vi "HoppingStep(Nonlinear-XZ-TargetModulation).vi"() -> ()   [LabVIEW 2014]
uses:
  <vilib>/Platform/TimedLoop/XDataNode/timing_clust.ctl
  <vilib>/Platform/TimedLoop/XDataNode/nitl_modes.ctl
  <vilib>/Platform/TimedLoop/XDataNode/wakeup.ctl
  <vilib>/rvi/Emulation/niFpgaGetClockAttributes.vi
  <vilib>/rvi/Emulation/niFpgaSctlEmulationGetInTimedLoop.vi
  <vilib>/rvi/Emulation/niFpgaEmulationReportErrorSimple.vi
  <vilib>/rvi/Emulation/niFpgaProcessEmulError.vi
  <vilib>/rvi/eio/common/nirviEmuTemplateMethod_errors.vi
  <vilib>/rvi/Emulation/niFpgaCriticalErrorInLSC.vi
  <vilib>/rvi/interface/RandomDataEmulation/niFpgaRandomDataHandleErrors.vi
  <vilib>/eio/EIONode/EIONode.xnode
  <vilib>/Platform/TimedLoop/XDataNode/XDataNode.xnode
  <vilib>/rvi/DataTransferAndStorage/Container/XNode/niFpgaContainer.xnode
  <vilib>/rvi/interface/RandomDataEmulation/nirviRandomDataFpgaReadWriteTemplate.vi
  <vilib>/Platform/TimedLoop/XDataNode/XDNodeRunTimeDep.lvlib
panel:
  in  "threshold":sgl
  in  "ExtraStepIn":u32
  in  "TimeConstant":u32
  in  "LowPassFilter":i16
  in  "BottomSleep us":i16=80
  in  "UpperSleep us":i16=150
  out "ZRealPos":i16
  in  "RelativeWithdraw":i16
  out "Waveform Chart":i32(graph)
  in  "stop":bool
  out "Z":i32(graph)
  in  "ZOffset":i16
  in  "XOffset":i16
  in  "XNum":i16
  in  "XStepIndex":i16
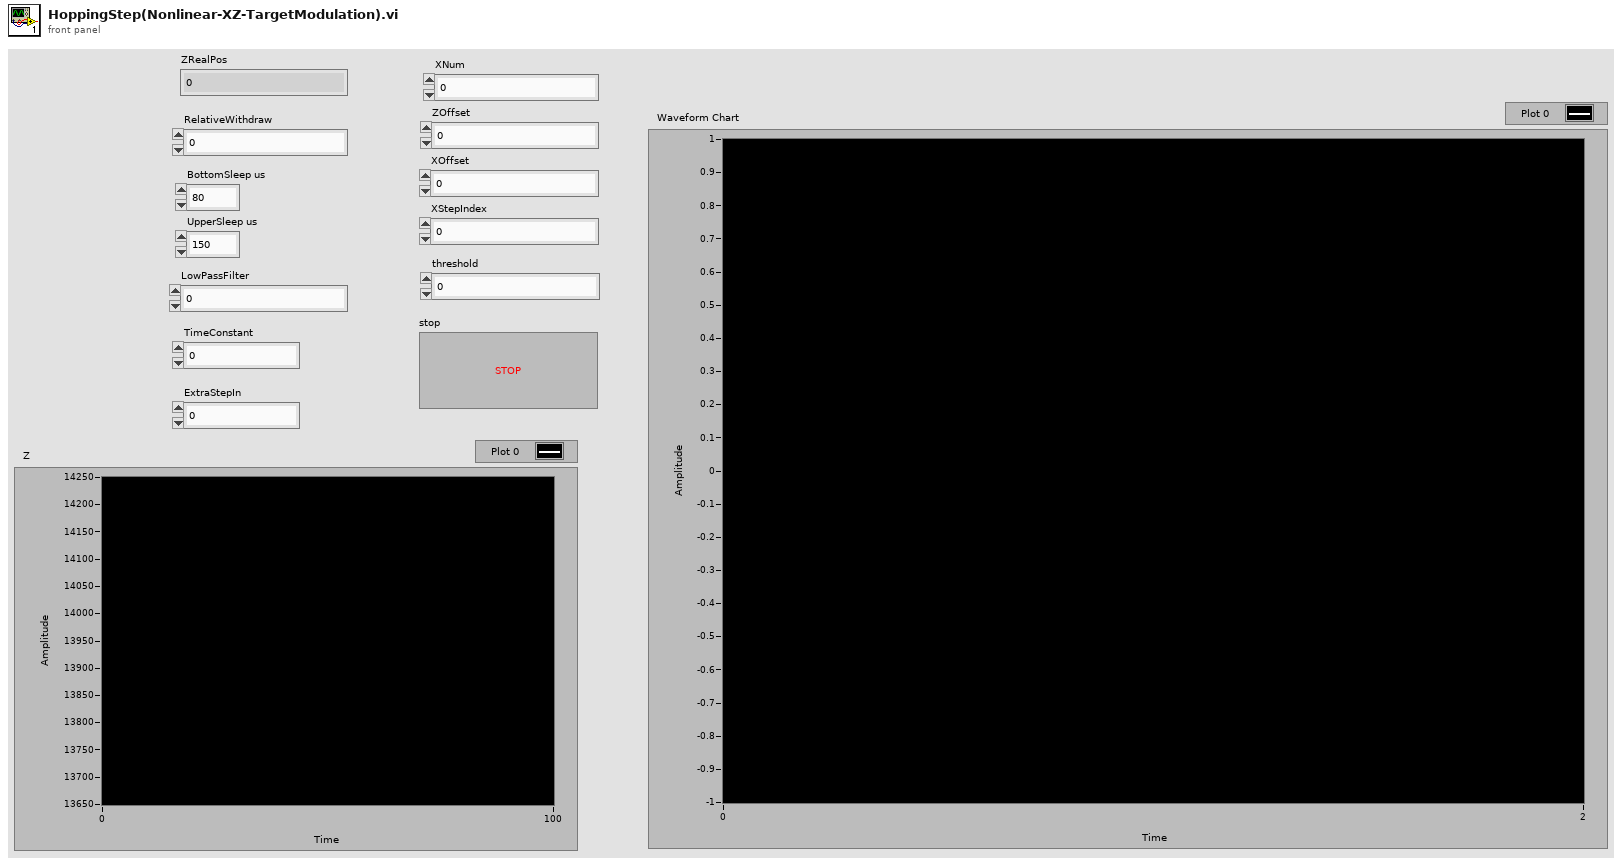
[diagram p1: front panel]
types:
  T1 = typedef "XDNodeRunTimeDep.lvlib/timing_clust.ctl" = cluster{"Expected End [f-1]":u64, "Actual End [f-1]":u64, "Finished Late? [f-1]":bool, "Expected End [i-1]":u64, "Actual End [i-1]":u64, "Finished Late? [i-1]":bool, "Expected Start [i]":u64, "Actual Start [i]":u64, "Expected Start [f]":u64, "Actual Start [f]":u64, "Source Name":string, "Structure Name":string, "Period":i64, "Deadline":i64, "Offset":i64, "Start":i64, "Priority":i32, "Timeout":i32, "Mode":T2, "Wakeup Reason":T3, "Error":errorcluster, "Source Type":string, "Secondary Source Type":string, "Global End Time":u64, "Global Start Time":u64, "Frame Duration":u64, "Iteration Duration":u64, "Assigned CPU":i32, "I/O Scan Engine Mode":u32}
  T2 = typedef "XDNodeRunTimeDep.lvlib/nitl_modes.ctl" = enum32{"No Change", "Process missed periods, maintain original phase", "Discard missed periods, maintain original phase", "Process missed periods, ignore original phase", "Discard missed periods, ignore original phase"}
  T3 = typedef "XDNodeRunTimeDep.lvlib/wakeup.ctl" = enum32{"Normal", "Aborted", "Asynchronous wakeup", "Timing source error", "Timed loop error", "Timeout"}
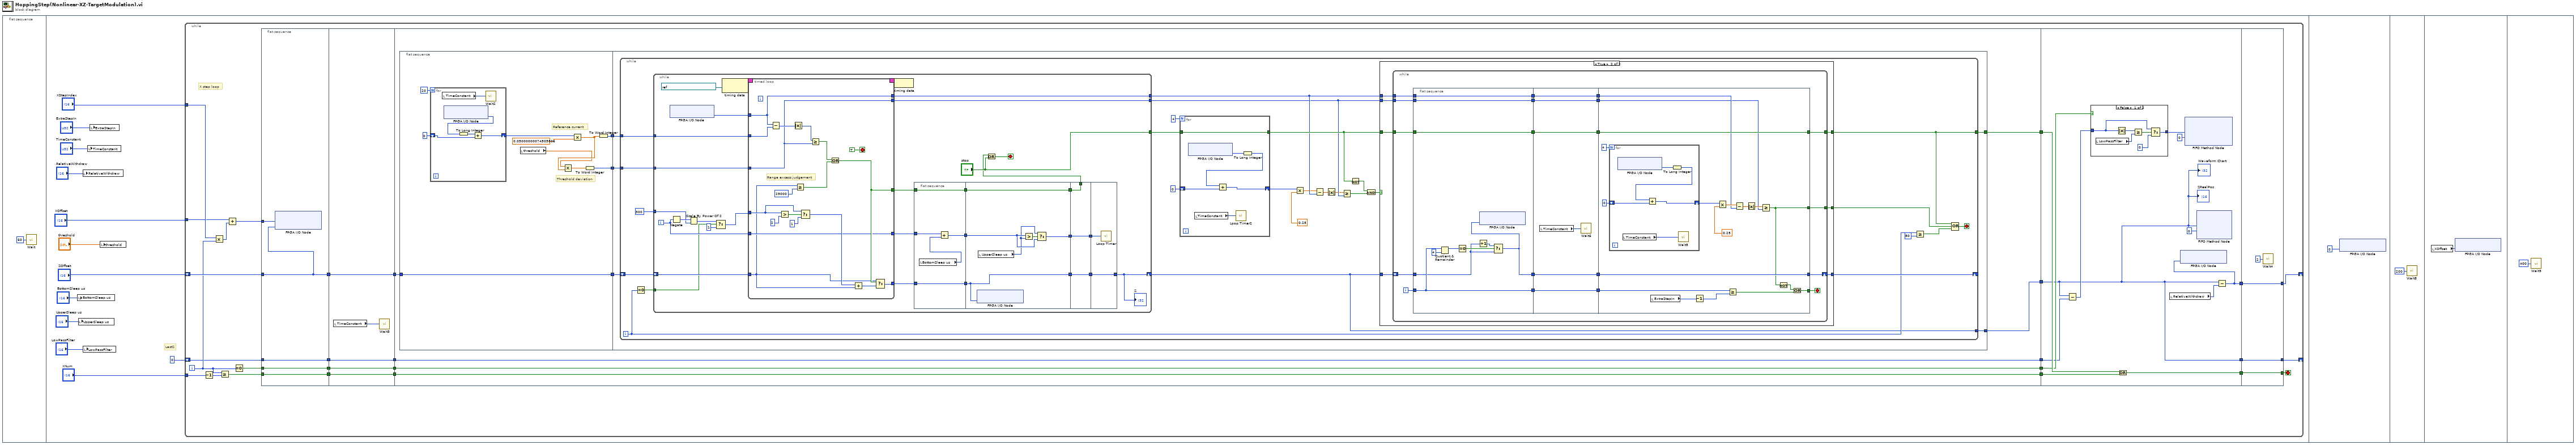
[diagram p0: block diagram]
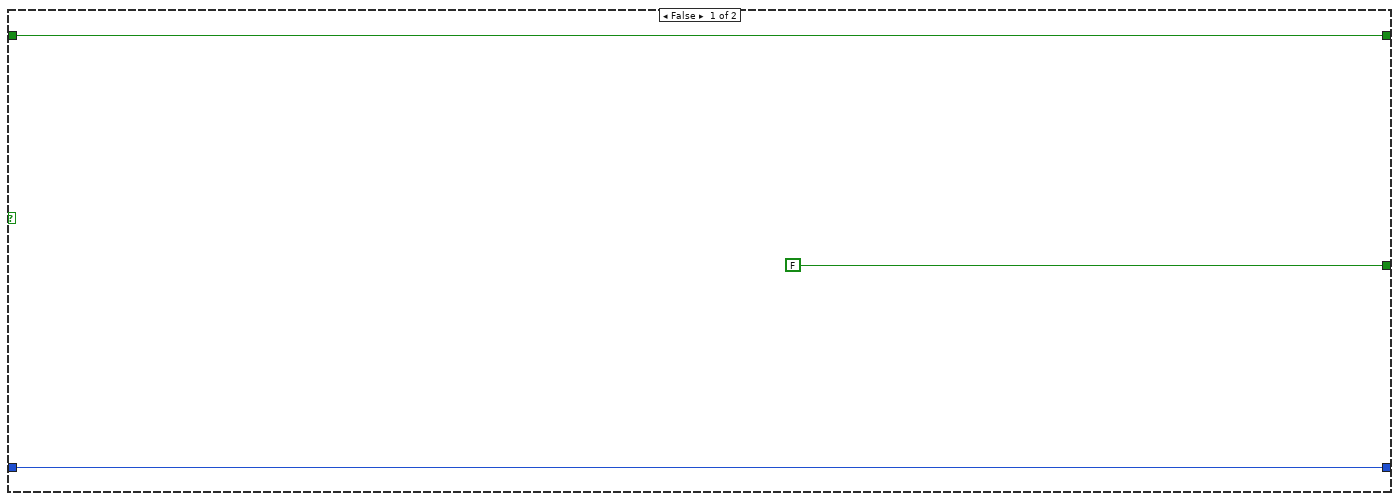
[diagram p2: hidden frame]
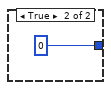
[diagram p3: hidden frame]
diagram:
  n1 = flat-sequence {
    frame #0 {
      n2 = call "Wait"("Count(mSec)"=u32 60 ("Count(uSec)")) -> ()  [unwired: 1 out]
    }
    frame #1 {
      # "LastZ"
      n3 = local write "BottomSleep us"("BottomSleep us") -> ()
      n4 = local write "UpperSleep us"("UpperSleep us") -> ()
      n5 = local write "RelativeWithdraw"("RelativeWithdraw") -> ()
      n6 = local write "LowPassFilter"("LowPassFilter") -> ()
      n7 = local write "TimeConstant"("TimeConstant") -> ()
      n8 = local write "ExtraStepIn"("ExtraStepIn") -> ()
      n9 = local write "threshold"("threshold") -> ()
      n10 = while {
        tunnel: "XNum" -> [w37]
        tunnel: "XStepIndex" -> [w38]
        shift-right: [w27] -> _
        shift-left: "ZOffset" -> [w39]
        tunnel: "XOffset" -> [w35]
        shift-right: [w17] -> _
        shift-left: i16 0 -> [w21]
        i -> [w26]
        stop <- w41 stop-if-true
        # "X step loop"
        n11 = Decrement(x=w37) -> (x-1=w36:i16)
        n12 = Multiply(x=w38, y=w26) -> (x*y=w40:i32)
        n13 = Greater Or Equal?(x=w26, y=w36) -> (x >= y?=w33:bool)
        n14 = Add(x=w35, y=w40) -> (x+y=w29:i32)
        n15 = Equal To 0?(x=w26) -> (x = 0?=w25:bool)
        n16 = flat-sequence {
          tunnel: [w48] -> w34
          tunnel: w39 -> [w48]
          tunnel: w33 -> [w47]
          tunnel: [w47] -> w31
          tunnel: w29 -> [w46]
          tunnel: w25 -> [w45]
          tunnel: [w45] -> w23
          tunnel: w21 -> [w44]
          tunnel: [w44] -> w19
          tunnel: [w53] -> w43
          tunnel: w34 -> [w53]
          tunnel: [w52] -> w32
          tunnel: w31 -> [w52]
          tunnel: [w51] -> w24
          tunnel: w23 -> [w51]
          tunnel: [w50] -> w20
          tunnel: w19 -> [w50]
          tunnel: w43 -> [w62]
          tunnel: [w61] -> w42
          tunnel: w32 -> [w60]
          tunnel: [w60] -> w30
          tunnel: [w54] -> w28
          tunnel: w24 -> [w56]
          tunnel: [w56] -> w22
          tunnel: w20 -> [w55]
          tunnel: [w55] -> w18
          tunnel: w42 -> [w265]
          tunnel: w30 -> [w264]
          tunnel: w28 -> [w257]
          tunnel: w22 -> [w262]
          tunnel: w18 -> [w258]
          tunnel: [w267] -> w16
          tunnel: [w256] -> w15
          tunnel: [w257] -> w14
          tunnel: [w276] -> w17
          tunnel: [w277] -> w27
          tunnel: [w278] -> w41
          tunnel: w16 -> [w278]
          tunnel: w15 -> [w277]
          tunnel: w14 -> [w276]
          frame #0 {
            n17 = xnode "FPGA I/O Node"("Connector0/AO2"=w46, "Connector0/AO0"=w48) -> ()  [unwired: 2 in, 2 out]
          }
          frame #1 {
            n18 = local read "TimeConstant"() -> (w49:u32)
            n19 = call "Wait3"("Count(uSec)"=w49) -> ()  [unwired: 1 out]
          }
          frame #2 {
            n20 = flat-sequence {
              tunnel: [w68] -> w59
              tunnel: [w69] -> w58
              tunnel: [w72] -> w57
              tunnel: w62 -> [w72]
              tunnel: [w82] -> w61
              tunnel: w59 -> [w81]
              tunnel: w58 -> [w80]
              tunnel: w57 -> [w79]
              tunnel: [w78] -> w54
              frame #0 {
                # "Threshold deviation"
                # "Reference current"
                n21 = for {
                  N: 20 -> [_]
                  shift-right: [w77] -> w67
                  shift-left: 0 -> [w76]
                  n22 = local read "TimeConstant"() -> (w73:u32)
                  n23 = xnode "FPGA I/O Node"() -> ("Connector0/AI1"=w74:i16)  [unwired: 1 in, 1 out]
                  n24 = To Long Integer(number=w74) -> (32bit integer=w75:i32)
                  n25 = Add(x=w75, y=w76) -> (x+y=w77:i32)
                  n26 = call "Wait2"("Count(uSec)"=w73) -> ()  [unwired: 1 out]
                }
                n27 = local read "threshold"() -> (w63:sgl)
                n28 = Multiply(x=w67, y=sgl 0.05) -> (x*y=w65:sgl)
                n29 = Multiply(x=w63, y=w65) -> (x*y=w70:sgl)
                n30 = To Word Integer(number=w70) -> (16bit integer=w69:i16)
                n31 = To Word Integer(number=w65) -> (16bit integer=w68:i16)
              }
              frame #1 {
                n32 = while {
                  tunnel: [w89] -> w82
                  tunnel: w81 -> [w95]
                  tunnel: w80 -> [w94]
                  shift-right: [w91] -> _
                  shift-left: w79 -> [w92]
                  tunnel: [w83] -> w78
                  i -> [w86]
                  stop <- w90 stop-if-true
                  n33 = Equal To 0?(x=w86) -> (x = 0?=w87:bool)
                  n34 = while {
                    tunnel: w95 -> [w133]
                    tunnel: w94 -> [w135]
                    tunnel: ["stop"] -> w103
                    shift-right: [w116] -> w83
                    shift-left: w92 -> [w130]
                    tunnel: i16 300 -> [w118]
                    tunnel: [w115] -> w107
                    tunnel: [w114] -> w106
                    tunnel: w87 -> [w113]
                    i -> [w117]
                    stop <- w137 stop-if-true
                    n35 = xnode "FPGA I/O Node"() -> ("Connector0/AI1"=w134:i16)  [unwired: 1 in, 1 out]
                    n36 = Negate(x=w117) -> (-x=w119:i32)
                    n37 = Scale By Power Of 2(n=w119, x=w118) -> (x*2^n=w112:i16)
                    n38 = Select(t=w112, s=w113, f=i16 1) -> (s? t:f=w110:i16)
                    n39 = node-c288(refnum<k21> "40 MHz Onboard Clock" ("Source Name")) -> (w140:T1)
                    n40 = timed-loop {
                      timing: w140 -> [_]
                      timing-out: [_] -> w139
                      tunnel: w133 -> [w174]
                      tunnel: w135 -> [w158]
                      tunnel: w134 -> [w157]
                      tunnel: [w170] -> w131
                      tunnel: [w169] -> w129
                      tunnel: w130 -> [w159]
                      tunnel: w110 -> [w162]
                      tunnel: [w164] -> w120
                      tunnel: w117 -> [w164]
                      tunnel: [w158] -> w114
                      tunnel: [w157] -> w115
                      stop <- TRUE stop-if-true
                      # "Range excess judgement"
                      n41 = Subtract(x=w157, y=w174) -> (x-y=w160:i16)
                      n42 = Greater?(x=w162, y=i16 2) -> (0:w161:bool)
                      n43 = Absolute Value(x=w160) -> (abs(x)=w173:i16)
                      n44 = Greater Or Equal?(x=w159, y=i16 29000) -> (x >= y?=w171:bool)
                      n45 = Select(t=w162, s=w161, f=1) -> (s? t:f=w165:i32)
                      n46 = Greater Or Equal?(x=w173, y=w158) -> (x >= y?=w172:bool)
                      n47 = Or(x=w172, y=w171) -> (x .or. y?=w169:bool)
                      n48 = Add(x=w165, y=w159) -> (x+y=w167:i32)
                      n49 = Select(t=w159, s=w169, f=w167) -> (s? t:f=w170:i32)
                    }
                    n50 = node-c288(w139) -> ()
                    n51 = flat-sequence {
                      tunnel: [w145] -> w132
                      tunnel: w131 -> [w145]
                      tunnel: w129 -> [w144]
                      tunnel: [w144] -> w128
                      tunnel: [w142] -> w121
                      tunnel: w120 -> [w143]
                      tunnel: w132 -> [w146]
                      tunnel: [w146] -> w127
                      tunnel: w128 -> [w151]
                      tunnel: [w151] -> w125
                      tunnel: [w149] -> w122
                      tunnel: w121 -> [w148]
                      tunnel: w127 -> [w154]
                      tunnel: [w154] -> w126
                      tunnel: w125 -> [w153]
                      tunnel: [w153] -> w124
                      tunnel: [w152] -> w123
                      tunnel: w122 -> [w152]
                      tunnel: w126 -> [w156]
                      tunnel: [w156] -> w116
                      tunnel: w123 -> [w155]
                      frame #0 {
                        n52 = local read "BottomSleep us"() -> (w141:i16)
                        n53 = Add(x=w143, y=w141) -> (x+y=w142:i32)
                      }
                      frame #1 {
                        n54 = xnode "FPGA I/O Node"("Connector0/AO0"=w146) -> ()  [unwired: 1 in, 1 out]
                        n55 = local read "UpperSleep us"() -> (w147:i16)
                        n56 = Greater?(x=w148, y=w147) -> (0:w150:bool)
                        n57 = Select(t=w147, s=w150, f=w148) -> (s? t:f=w149:i32)
                      }
                      frame #2 {
                      }
                      frame #3 {
                        n58 = call "Loop Timer"("Count(uSec)"=w155) -> ()  [unwired: 1 out]
                      }
                    }
                    n59 = Or(x=w124, y="stop") -> (x .or. y?=w137:bool)
                    "Z" <- w116
                  }
                  n60 = for {
                    N: 4 -> [_]
                    tunnel: w103 -> [w187]
                    tunnel: [w187] -> w108
                    shift-right: [w183] -> w101
                    shift-left: 0 -> [w185]
                    n61 = xnode "FPGA I/O Node"() -> ("Connector0/AI1"=w186:i16)  [unwired: 1 in, 1 out]
                    n62 = local read "TimeConstant"() -> (w182:u32)
                    n63 = call "Loop Timer2"("Count(uSec)"=w182) -> ()  [unwired: 1 out]
                    n64 = To Long Integer(number=w186) -> (32bit integer=w184:i32)
                    n65 = Add(x=w184, y=w185) -> (x+y=w183:i32)
                  }
                  n66 = Multiply(x=w101, y=sgl 0.25) -> (x*y=w100:sgl)
                  n67 = Subtract(x=w100, y=w107) -> (x-y=w99:sgl)
                  n68 = Absolute Value(x=w99) -> (abs(x)=w98:sgl)
                  n69 = Greater Or Equal?(x=w98, y=w106) -> (x >= y?=w97:bool)
                  n70 = Not(x=w108) -> (.not. x?=w96:bool)
                  n71 = And(x=w96, y=w97) -> (x .and. y?=w109:bool)
                  n72 = case shown="True" w109 {
                    tunnel: w108 -> [w190 w197]
                    tunnel: [w190 w196] -> w89
                    tunnel: w107 -> [_ w195]
                    tunnel: w106 -> [_ w194]
                    tunnel: w83 -> [w189 w193]
                    tunnel: [w189 w192] -> w91
                    tunnel: [FALSE w191] -> w88
                    frame False {
                    }
                    frame True {
                      n73 = while {
                        tunnel: w195 -> [w206]
                        tunnel: w194 -> [w205]
                        tunnel: [w202] -> w191
                        shift-right: [w203] -> w192
                        shift-left: w193 -> [w204]
                        tunnel: w197 -> [w208]
                        tunnel: [w207] -> w196
                        i -> [w200]
                        stop <- w198 stop-if-true
                        n74 = flat-sequence {
                          tunnel: w205 -> [w224]
                          tunnel: w206 -> [w225]
                          tunnel: w208 -> [w226]
                          tunnel: [w226] -> w216
                          tunnel: [w225] -> w215
                          tunnel: [w224] -> w214
                          tunnel: w204 -> [w218]
                          tunnel: [w217] -> w213
                          tunnel: [w223] -> w201
                          tunnel: w200 -> [w223]
                          tunnel: [w232] -> w212
                          tunnel: [w231] -> w211
                          tunnel: [w230] -> w210
                          tunnel: w216 -> [w232]
                          tunnel: w215 -> [w231]
                          tunnel: w214 -> [w230]
                          tunnel: [w229] -> w209
                          tunnel: w213 -> [w229]
                          tunnel: w201 -> [w227]
                          tunnel: [w227] -> w199
                          tunnel: w212 -> [w250]
                          tunnel: [w250] -> w207
                          tunnel: w211 -> [w242]
                          tunnel: w210 -> [w241]
                          tunnel: w209 -> [w240]
                          tunnel: [w240] -> w203
                          tunnel: [w234] -> w202
                          tunnel: w199 -> [w239]
                          tunnel: [w235] -> w198
                          frame #0 {
                            n75 = Quotient & Remainder(x=w223, y=4) -> (x-y*floor(x/y)=w221:i32)  [unwired: 1 out]
                            n76 = Equal To 0?(x=w221) -> (x = 0?=w220:bool)
                            n77 = Increment(x=w218) -> (x+1=w219:i32)
                            n78 = Select(t=w219, s=w220, f=w218) -> (s? t:f=w217:i32)
                            n79 = xnode "FPGA I/O Node"("Connector0/AO0"=w217) -> ()  [unwired: 1 in, 1 out]
                          }
                          frame #1 {
                            n80 = local read "TimeConstant"() -> (w228:u32)
                            n81 = call "Wait6"("Count(uSec)"=w228) -> ()  [unwired: 1 out]
                          }
                          frame #2 {
                            n82 = for {
                              N: 4 -> [_]
                              shift-right: [w252] -> w247
                              shift-left: 0 -> [w254]
                              n83 = xnode "FPGA I/O Node"() -> ("Connector0/AI1"=w255:i16)  [unwired: 1 in, 1 out]
                              n84 = local read "TimeConstant"() -> (w251:u32)
                              n85 = To Long Integer(number=w255) -> (32bit integer=w253:i32)
                              n86 = Add(x=w253, y=w254) -> (x+y=w252:i32)
                              n87 = call "Wait5"("Count(uSec)"=w251) -> ()  [unwired: 1 out]
                            }
                            n88 = local read "ExtraStepIn"() -> (w238:u32)
                            n89 = Decrement(x=w238) -> (x-1=w237:u32)
                            n90 = Multiply(x=w247, y=sgl 0.25) -> (x*y=w244:sgl)
                            n91 = Greater Or Equal?(x=w239, y=w237) -> (x >= y?=w236:bool)
                            n92 = Subtract(x=w244, y=w242) -> (x-y=w245:sgl)
                            n93 = Absolute Value(x=w245) -> (abs(x)=w243:sgl)
                            n94 = Greater Or Equal?(x=w243, y=w241) -> (x >= y?=w234:bool)
                            n95 = Not(x=w234) -> (.not. x?=w233:bool)
                            n96 = Or(x=w233, y=w236) -> (x .or. y?=w235:bool)
                          }
                        }
                      }
                    }
                  }
                  n97 = Greater Or Equal?(x=w86, y=80) -> (x >= y?=w84:bool)
                  n98 = Compound Arithmetic op=OR(w89, w88, w84) -> (w90:bool)
                }
              }
            }
          }
          frame #3 {
            n99 = Subtract(x=w257, y=w258) -> (x-y=w259:i32)
            n100 = case shown="False" w262 {
              tunnel: w259 -> [w269 _]
              tunnel: [w270 0 ("f")] -> w261
              frame False {
                n101 = local read "LowPassFilter"() -> (w272:i16)
                n102 = Absolute Value(x=w269) -> (abs(x)=w268:i32)
                n103 = Greater Or Equal?(x=w268, y=w272) -> (x >= y?=w273:bool)
                n104 = Select(t=w269, s=w273, f=0) -> (s? t:f=w270:i32)
              }
              frame True {
              }
            }
            n105 = Or(x=w265, y=w264) -> (x .or. y?=w267:bool)
            n106 = local read "RelativeWithdraw"() -> (w263:i16)
            n107 = xnode ("FIFO Method Node")("Element"=w261, "Timeout"=0) -> ()  [unwired: 1 in, 2 out]
            n108 = xnode ("FIFO Method Node")("Element"=w257, "Timeout"=0) -> ()  [unwired: 1 in, 2 out]
            n109 = Subtract(x=w257, y=w263) -> (x-y=w256:i32)
            n110 = xnode "FPGA I/O Node"("Connector0/AO0"=w256) -> ()  [unwired: 1 in, 1 out]
            "Waveform Chart" <- w257
            "ZRealPos" <- w257
          }
          frame #4 {
            n111 = call "Wait4"("Count(mSec)"=u32 2) -> ()  [unwired: 1 out]
          }
        }
      }
    }
    frame #2 {
      n112 = xnode "FPGA I/O Node"("Connector0/AO0"=i16 0) -> ()  [unwired: 1 in, 1 out]
    }
    frame #3 {
      n113 = call "Wait8"("Count(uSec)"=u32 200) -> ()  [unwired: 1 out]
    }
    frame #4 {
      n114 = local read "XOffset"() -> (w281:i16)
      n115 = xnode "FPGA I/O Node"("Connector0/AO2"=w281) -> ()  [unwired: 1 in, 1 out]
    }
    frame #5 {
      n116 = call "Wait9"("Count(uSec)"=u32 400) -> ()  [unwired: 1 out]
    }
  }
